vi "jsontest.vi"(8 "error in (no error)":errorcluster, 11 "string":string="This is posted to #patcherBot_status and comes from *monkey-bot*.") -> (0 "error out":errorcluster)   [LabVIEW 2019]
uses:
  <vilib>/httpClient/POSTBuffer.vi
  <vilib>/httpClient/LabVIEWHTTPClient.lvlib
panel:
  out "headers":string
  out "body":string
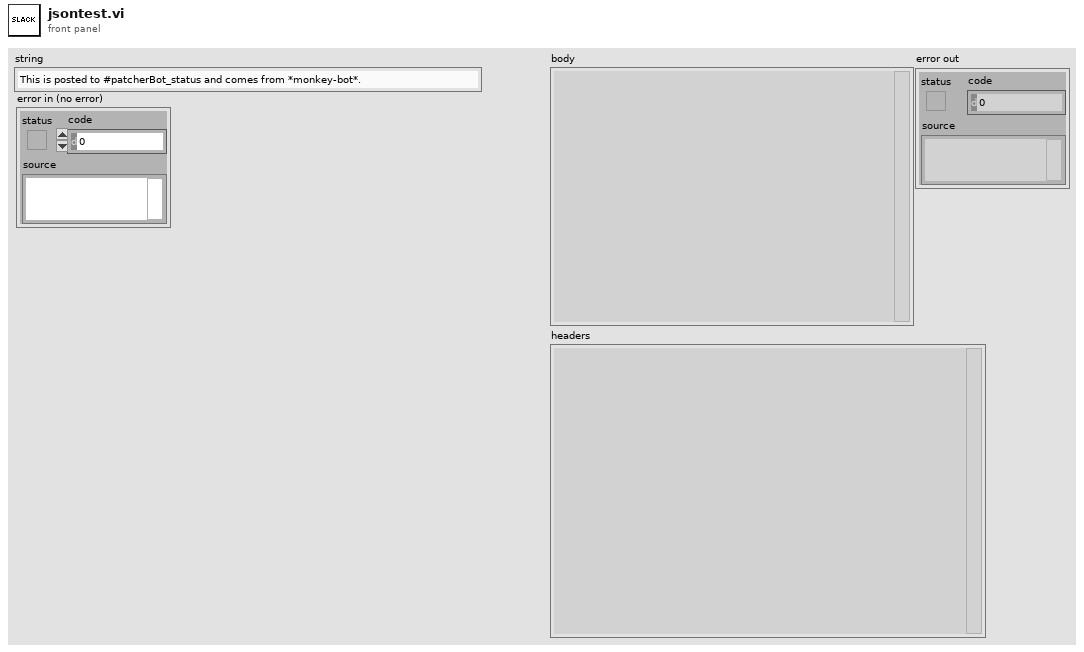
[diagram p1: front panel]
types:
  T1 = typedef "LabVIEWHTTPClient.lvlib/ClientHandle.ctl" = refnum<k1>
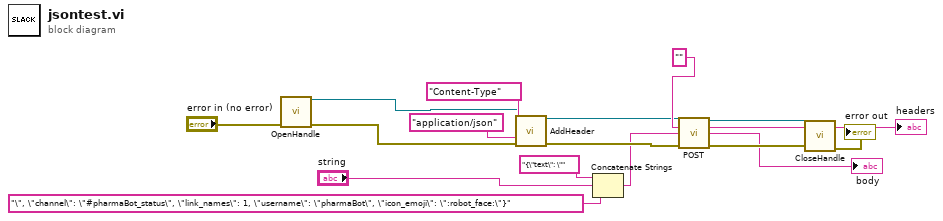
[diagram p0: block diagram]
diagram:
  n1 = call <vilib>:"OpenHandle.vi"("error in (no error)"="error in (no error)") -> ("client handle out"=w11:T1, "error out"=w10:errorcluster)  [unwired: 13 in]
  n2 = call <vilib>:"AddHeader.vi"("client handle"=w11, "header"="Content-Type", "value"="application/json", "error in (no error)"=w10) -> ("client handle out"=w7:T1, "error out"=w14:errorcluster)  [unwired: 10 in]
  n3 = Concatenate Strings("{\"text\": \"" ("string"), "string", "\", \"channel\": \"#pharmaBot_status\", \"link_names\": 1, \"username\": \"pharmaBot\", \"icon_emoji\": \":robot_face:\"}" ("string")) -> (w3:string)
  n4 = call-poly <vilib>:"POST.vi"("client handle"=w7, "url"="", "buffer"=w3, "error in (no error)"=w14) -> ("client handle out"=w16:T1, "headers"=→"headers":string, "body"=→"body":string, "error out"=w17:errorcluster)  [unwired: 8 in]
  n5 = call <vilib>:"CloseHandle.vi"("client handle"=w16, "error in (no error)"=w17) -> ("error out"=→"error out":errorcluster)  [unwired: 13 in]
